vi "Configure Temperature User RTD.vi"(6 "Zero":dbl=100.0, 7 "Delta":dbl=1.4999, 8 "error in (no error)":errorcluster, 9 "Beta":dbl=0.10863, 10 "Alpha":dbl=0.0038506, 11 "VISA resource name":refnum<visa-resource-name>) -> (0 "error out":errorcluster, 3 "VISA resource name out":refnum<visa-resource-name>)   [LabVIEW 2025, in "Keithley DMM7510.lvlib"]
doc: "This VI configues the Alpha, Beta, Delta and Zero values for user defined RTD that is being used."
uses:
  Keithley DMM7510.lvlib
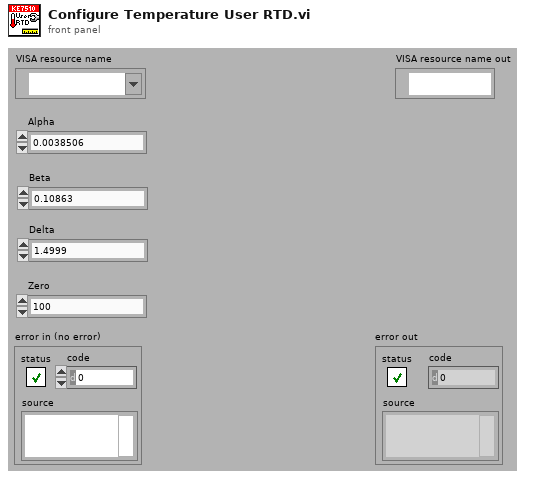
[diagram p1: front panel]
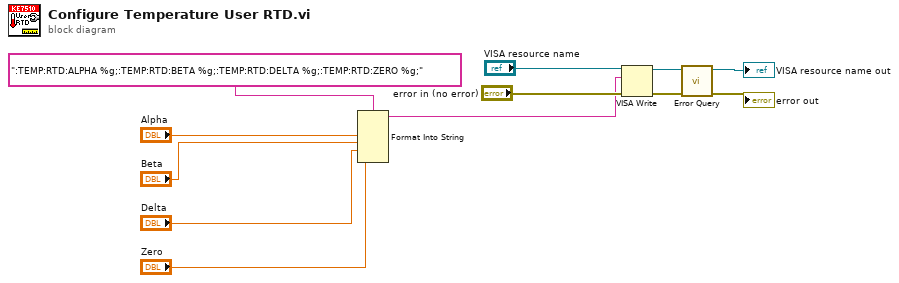
[diagram p0: block diagram]
diagram:
  n1 = Format Into String(format string=":TEMP:RTD:ALPHA %g;:TEMP:RTD:BETA %g;:TEMP:RTD:DELTA %g;:TEMP:RTD:ZERO %g;", "Alpha", "Beta", "Delta", "Zero") -> (resulting string=w5:string)  [unwired: 2 in, 1 out]
  n2 = VISA Write(VISA resource name="VISA resource name", write buffer=w5, error in (no error)="error in (no error)") -> (VISA resource name out=w9:refnum<visa-resource-name>, error out=w8:errorcluster)  [unwired: 1 out]
  n3 = call "Error Query.vi"("error in (no error)"=w8, "VISA resource name"=w9) -> ("error out"=→"error out":errorcluster, "VISA resource name out"=→"VISA resource name out":refnum<visa-resource-name>)  [unwired: 6 in, 2 out]
